vi "Bring to Front.vi"(8 "error in (no error)":errorcluster, 11 "Excel Interface in":refnum<class "Excel Interface.lvclass">) -> (0 "error out":errorcluster, 3 "Excel Interface out":refnum<class "Excel Interface.lvclass">)   [LabVIEW 2016, in "Excel Interface.lvclass"]
uses:
  Excel Interface.lvclass
  user32.dll
panel:
  out "Excel._Application":refnum<k7>
  in  "error in":errorcluster
  in  "Excel._Application 2":refnum<k7>
  out "error out 2":errorcluster
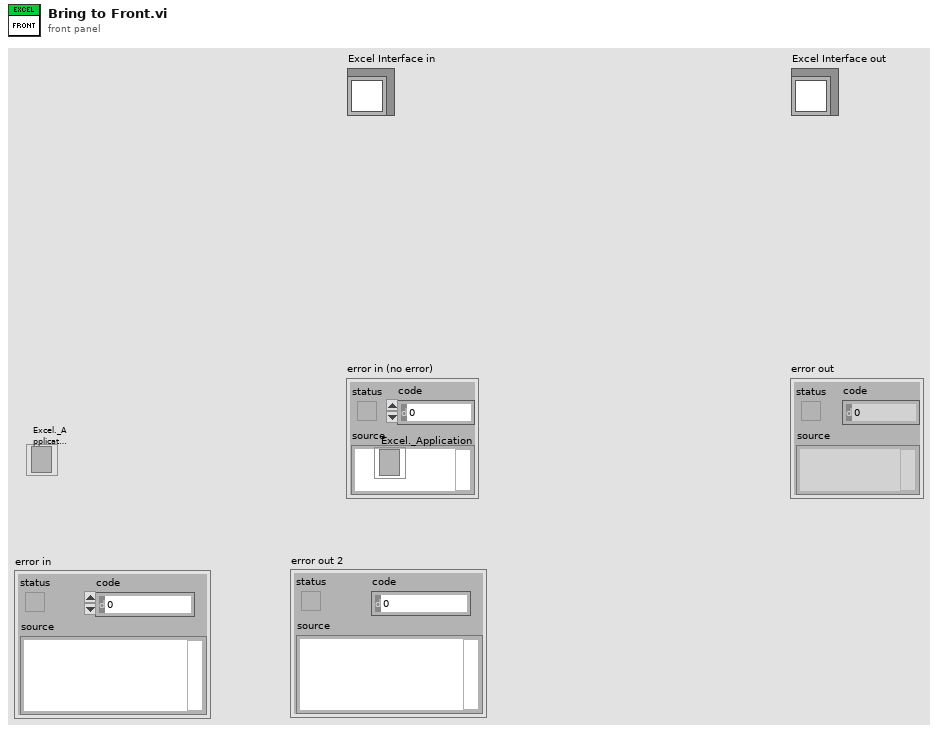
[diagram p1: front panel]
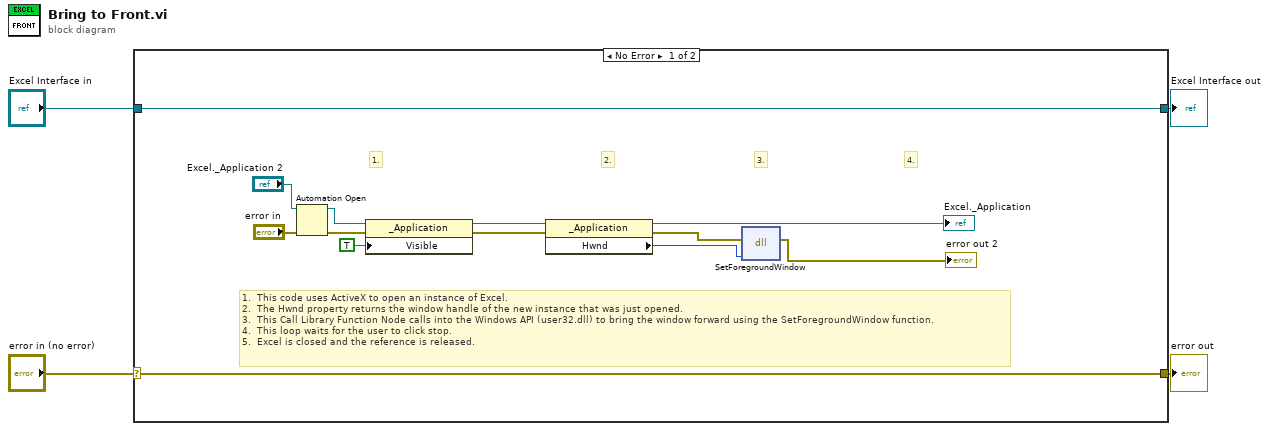
[diagram p0: block diagram]
diagram:
  n1 = case shown="No Error" "error in (no error)" {
    selector: "error in (no error)" -> [w16 w19]
    tunnel: [w16 w19] -> w3
    tunnel: [w17 w18] -> w1
    tunnel: "Excel Interface in" -> [w17 w18]
    frame No Error {
      # "1.  This code uses ActiveX to open an instance of Excel.\n2.  The Hwnd property returns the window handle of the new instance that was just opened.\n3.  This Call Library Function Node calls into the Windows API (user32.dll) to bring the window forward using the SetForegroundWindow function.\n4.  This loop waits for the user to click stop.\n5.  Excel is closed and the reference is released."
      # "3."
      # "4."
      # "2."
      # "1."
      n2 = Automation Open(error in (no error)="error in", Automation Refnum="Excel._Application 2") -> (Automation Refnum=w7:refnum<k7>, error out=w8:errorcluster)  [unwired: 2 in]
      n3 = property class="_Application"(reference=w7, error in=w8, "Visible"=TRUE) -> (reference out=w10:refnum<k7>, error out=w9:errorcluster)
      n4 = property class="_Application"(reference=w10, error in=w9) -> (reference out=→"Excel._Application":refnum<k7>, error out=w12:errorcluster, "Hwnd"=w14:i32)
      n5 = dll-call lib="user32.dll" fn="SetForegroundWindow"(error in=w12, "Handle"=w14) -> (error out=→"error out 2":errorcluster)  [unwired: 3 in, 2 out]
    }
    frame Error {
    }
  }
  "error out" <- w3
  "Excel Interface out" <- w1
